vi "Enable Current Sharing.vi"(8 "error in (no error)":errorcluster, 11 "69X_79X in":refnum<class "69X_79X.lvclass">) -> (0 "error out":errorcluster, 3 "69X_79X out":refnum<class "69X_79X.lvclass">)   [LabVIEW 2019, in "69X_79X.lvlib" / "69X_79X.lvclass"]
uses:
  Library/69X_79X.lvclass
  C:/Users/Public/Documents/Development/builds/Instruments/PowerSupply.lvlibp/Library/PowerSupply.lvclass
  Library/69X_79X.lvclass/69X_79X.ctl
  Accessors/Read Local Resource.vi
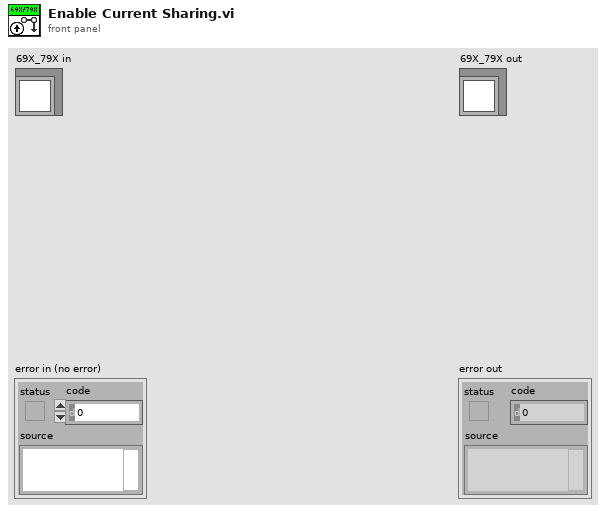
[diagram p1: front panel]
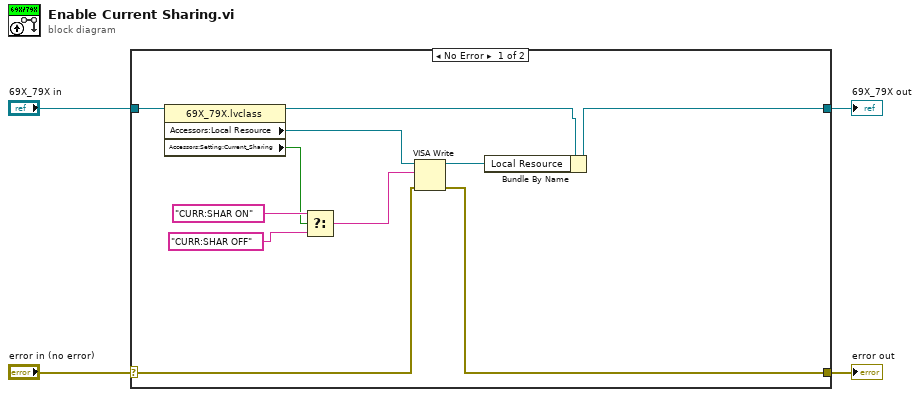
[diagram p0: block diagram]
diagram:
  n1 = case shown="No Error" "error in (no error)" {
    selector: "error in (no error)" -> [w13 w17]
    tunnel: [w12 w17] -> w3
    tunnel: [w15 w16] -> w1
    tunnel: "69X_79X in" -> [w11 w16]
    frame No Error {
      n2 = property class="69X_79X.lvclass"(reference=w11) -> (reference out=w10:refnum<class "69X_79X.lvclass">, "Accessors:Local Resource"=w9:refnum<visa-resource-name>, "Accessors:Setting:Current_Sharing"=w6:bool)  [unwired: 1 in, 1 out]
      n3 = Select(t="CURR:SHAR ON" ("write buffer"), s=w6, f="CURR:SHAR OFF" ("write buffer")) -> (s? t:f=w7:string)
      n4 = VISA Write(VISA resource name=w9, write buffer=w7, error in (no error)=w13) -> (VISA resource name out=w14:refnum<visa-resource-name>, error out=w12:errorcluster)  [unwired: 1 out]
      n5 = Bundle By Name(cluster=w10, "Local Resource"=w14) -> (w15:refnum<class "69X_79X.lvclass">)
    }
    frame Error {
    }
  }
  "error out" <- w3
  "69X_79X out" <- w1
